vi "Write.Initialize.vi"(8 "error in (no error)":errorcluster, 11 "Settings":cluster{"Refs":T1[], "Values":dbl[]} {"Refs" format="%.0x"}) -> (0 "error out":errorcluster, 3 "Write out":refnum<class "Write.lvclass">)   [LabVIEW 2015, in "Data Access Engine.lvlib" / "Write.lvclass"]
uses:
  Write.lvclass
  <vilib>/NI Veristand/Custom Device API/Data Reference.ctl
  Write.lvclass/Write.ctl
  <vilib>/NI Veristand/Custom Device API/Custom Device API.lvlib
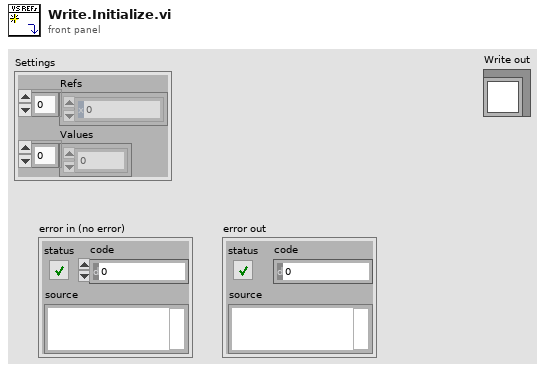
[diagram p1: front panel]
types:
  T1 = typedef "Custom Device API.lvlib/Data Reference.ctl" = i32
  T2 = cluster{"read mode":enum16{"polling", "blocking"}, "write mode":enum16{"polling", "blocking"}}
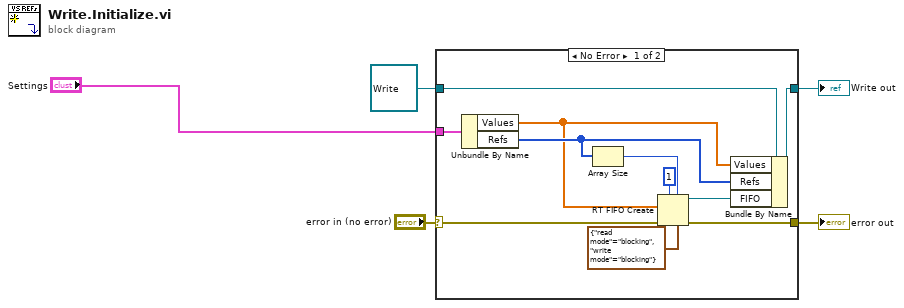
[diagram p0: block diagram]
diagram:
  n1 = case shown="No Error" "error in (no error)" {
    selector: "error in (no error)" -> [w9 w17]
    tunnel: [w16 w17] -> w5
    tunnel: refnum<class "Write.lvclass"> refnum ("Write in") -> [w11 w18]
    tunnel: [w10 w18] -> w3
    tunnel: "Settings" -> [w8 _]
    frame No Error {
      n2 = Unbundle By Name(w8) -> ("Values"=w6:dbl[], "Refs"=w7:T1[])
      n3 = Array Size(array=w7) -> (size(s)=w13:i32)
      n4 = RT FIFO Create(1:w6, 3:w9, 4:u32 1 ("size (10)"), 6:w13, 7:T2 {"read mode"=enum."blocking", "write mode"=enum."blocking"} ("r/w modes (polling,polling)")) -> (8:w15:refnum<k33>, 11:w16:errorcluster)  [unwired: 3 in, 1 out]
      n5 = Bundle By Name(cluster=w11, "Values"=w6, "Refs"=w7, "FIFO"=w15) -> (w10:refnum<class "Write.lvclass">)
    }
    frame Error {
    }
  }
  "error out" <- w5
  "Write out" <- w3
